vi "manual control.vi"(8 "error in (no error)":errorcluster, 10 "control":T1={"Pump Direction"=0, "Flow rate (ml/min)"=1.0, "Target volum (ml)"=1.0, "Run"=FALSE} {"Target volum (ml)" format="%#.4f"; "Flow rate (ml/min)" format="%#.4f"; "Pump Direction" items=["Infuse", "Withdraw"]}, 11 "VISA resource name":refnum<visa-resource-name>) -> (0 "error out":errorcluster, 3 "VISA resource name out":refnum<visa-resource-name>)   [LabVIEW 2017]
uses:
  <instrlib>/Harvard Apparatus PHD Ultra Series/Harvard Apparatus PHD Ultra Series.lvlib
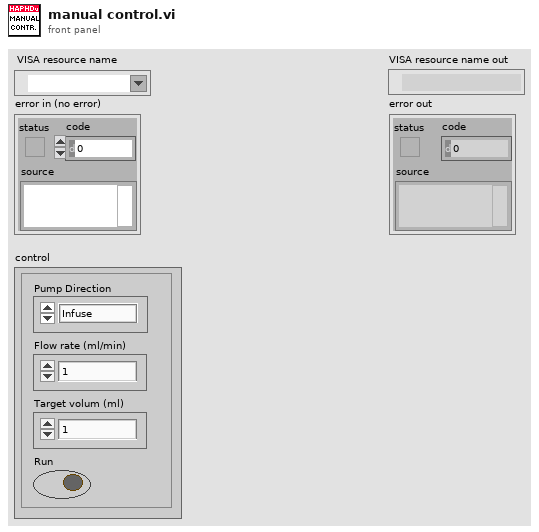
[diagram p1: front panel]
types:
  T1 = cluster{"Pump Direction":u16, "Flow rate (ml/min)":dbl, "Target volum (ml)":dbl, "Run":bool}
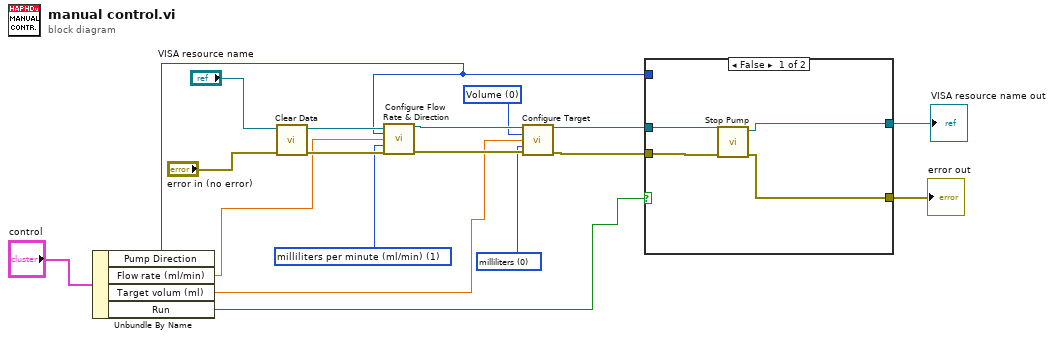
[diagram p0: block diagram]
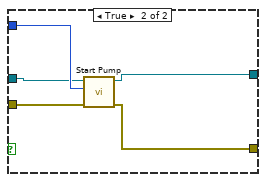
[diagram p2: hidden frame]
diagram:
  w8 = u16 0 items=["Volume", "Time"] ("Target Type (0:Volume)")
  w9 = u16 0 items=["milliliters", "microliters", "nanoliters", "picoliters"] ("Volume Units (0:ml)")
  w10 = u32 1 items=["milliliters per hour (ml/hr)", "milliliters per minute (ml/min)", "milliliters per second (ml/sec)", "microliters per hour (ul/hr)", "microliters per minute (ul/min)", "microliters per second (ul/sec)", "nanoliters per hour (nl/hr)", "nanoliters per minute (nl/min)", "nanoliters per second (nl/sec)", "picoliters per hour (pl/hr)", "picoliters per minute (pl/min)", "picoliters per second (pl/sec)"] ("Flow Rate Units (1:ml/min)")
  n1 = Unbundle By Name("control") -> ("Pump Direction"=w1:u16, "Flow rate (ml/min)"=w3:dbl, "Target volum (ml)"=w2:dbl, "Run"=w4:bool)
  n2 = call <instrlib>:"Clear Data.vi"("error in (no error)"="error in (no error)", "VISA resource name"="VISA resource name") -> ("error out"=w17:errorcluster, "VISA resource name out"=w18:refnum<visa-resource-name>)  [unwired: 8 in]
  n3 = call <instrlib>:"Configure Flow Rate & Direction.vi"("VISA resource name"=w18, "Pump Direction (0:Infuse)"=w1, "Flow Rate (5.00)"=w3, "Flow Rate Units (1:ml/min)"=w10, "error in (no error)"=w17) -> ("VISA resource name out"=w13:refnum<visa-resource-name>, "error out"=w16:errorcluster)  [unwired: 9 in]
  n4 = call <instrlib>:"Configure Target.vi"("VISA resource name"=w13, "Target Type (0:Volume)"=w8, "Target Value (5.00)"=w2, "Volume Units (0:ml)"=w9, "error in (no error)"=w16) -> ("VISA resource name out"=w14:refnum<visa-resource-name>, "error out"=w15:errorcluster)  [unwired: 9 in]
  n5 = case shown="False" w4 {
    tunnel: w15 -> [w22 w25]
    tunnel: w14 -> [w21 w26]
    tunnel: w1 -> [_ w27]
    tunnel: [w20 w24] -> w7
    tunnel: [w19 w23] -> w6
    frame False {
      n6 = call <instrlib>:"Stop Pump.vi"("error in (no error)"=w22, "VISA resource name"=w21) -> ("error out"=w19:errorcluster, "VISA resource name out"=w20:refnum<visa-resource-name>)  [unwired: 8 in]
    }
    frame True {
      n7 = call <instrlib>:"Start Pump.vi"("error in (no error)"=w25, "Run Direction (0:Infuse)"=w27, "VISA resource name"=w26) -> ("error out"=w23:errorcluster, "VISA resource name out"=w24:refnum<visa-resource-name>)  [unwired: 7 in]
    }
  }
  "VISA resource name out" <- w7
  "error out" <- w6
